vi "Normalizesignal.vi"(5 "Yoffset":sgl, 6 "sum_offset":sgl, 7 "Xoffset":sgl, 8 "Normalize signal":bool, 9 "Sum":sgl, 10 "Y":sgl, 11 "X":sgl) -> (1 "Sum":sgl, 2 "Y":sgl, 3 "X":sgl)   [LabVIEW 2019]
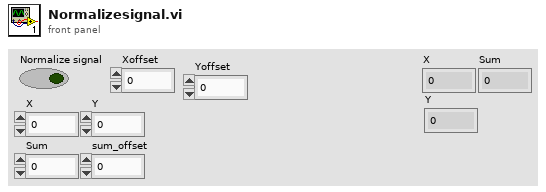
[diagram p1: front panel]
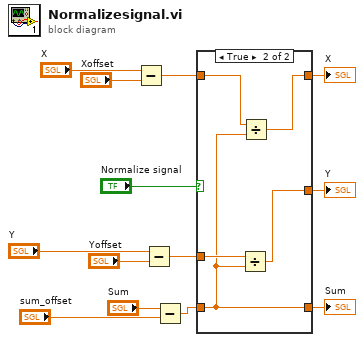
[diagram p0: block diagram]
diagram:
  n1 = Subtract(x="X", y="Xoffset") -> (x-y=w4:sgl)
  n2 = Subtract(x="Y", y="Yoffset") -> (x-y=w1:sgl)
  n3 = Subtract(x="Sum", y="sum_offset") -> (x-y=w8:sgl)
  n4 = case shown="True" "Normalize signal" {
    tunnel: w1 -> [w15 w21]
    tunnel: w8 -> [w14 w17]
    tunnel: w4 -> [w16 w20]
    tunnel: [w16 w19] -> w12
    tunnel: [w14 w17] -> w10
    tunnel: [w15 w18] -> w11
    frame False {
    }
    frame True {
      n5 = Divide(x=w21, y=w17) -> (x/y=w18:sgl)
      n6 = Divide(x=w20, y=w17) -> (x/y=w19:sgl)
    }
  }
  "X" <- w12
  "Y" <- w11
  "Sum" <- w10
